vi "CMN_LabMathParser.vi"(8 "error in (no error)":errorcluster, 9 "expression":string="x", 10 "x":dbl format="%.2f") -> (0 "error out":errorcluster, 2 "answer":dbl format="%.2f")   [LabVIEW 2016]
uses:
  <vilib>/gmath/NI_Gmath.lvlib
panel:
  out "err":i32
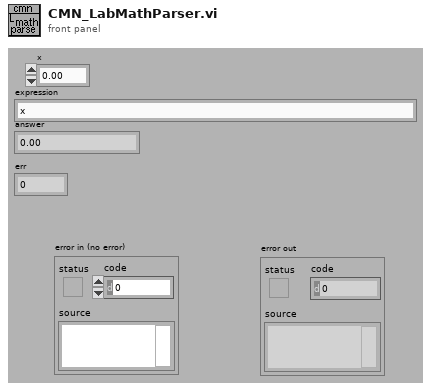
[diagram p1: front panel]
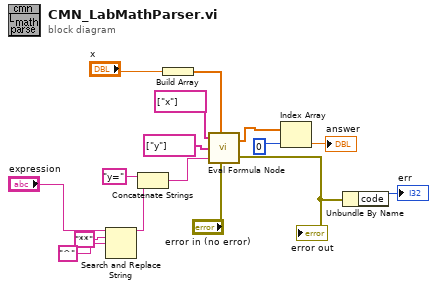
[diagram p0: block diagram]
diagram:
  n1 = Search and Replace String(input string="expression", search string="**", replace string="^" ("replace string (\"\")")) -> (result string=w2:string)  [unwired: 1 in, 7 out]
  n2 = Concatenate Strings("y=" ("string"), w2) -> (w11:string)
  n3 = Build Array("x") -> (w13:dbl[])
  n4 = call <vilib>:"Eval Formula Node.vi"("Variables Input"=string[] ["x"], "Input Values"=w13, "Variables Output"=string[] ["y"], "formula"=w11, "error in (no error)"="error in (no error)") -> ("Output Values"=w9:dbl[], "error out"=w6:errorcluster)
  "error out" <- w6
  n5 = Index Array(array=w9, index=0) -> (element=→"answer":dbl)
  n6 = Unbundle By Name(w6) -> ("code"=→"err":i32)
